vi "InitWaveforms.vi"(6 "First Read":bool, 7 "Samples Per Channel":i32, 8 "error in (no error)":errorcluster, 9 "Sample Rate":dbl, 10 "Units":string[](array[string]), 11 "Channels":string[](array[string])) -> (0 "error out":errorcluster, 3 "wfm array":waveform(sgl)[](array[waveform]))   [LabVIEW 2017, in "cRIOWfmLib.lvlib"]
uses:
  <vilib>/addons/InsightCM/Devices/Shared/Cms/cRIOWfmAcq/cRIOWfmLib.lvlib
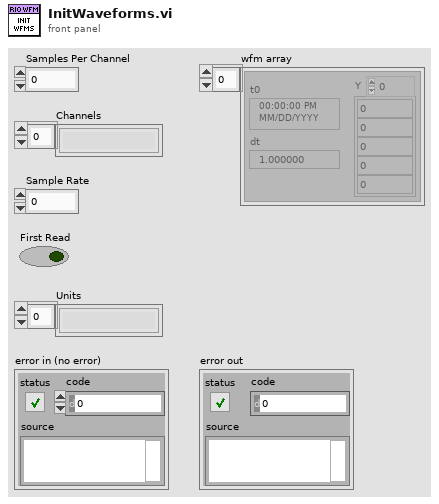
[diagram p1: front panel]
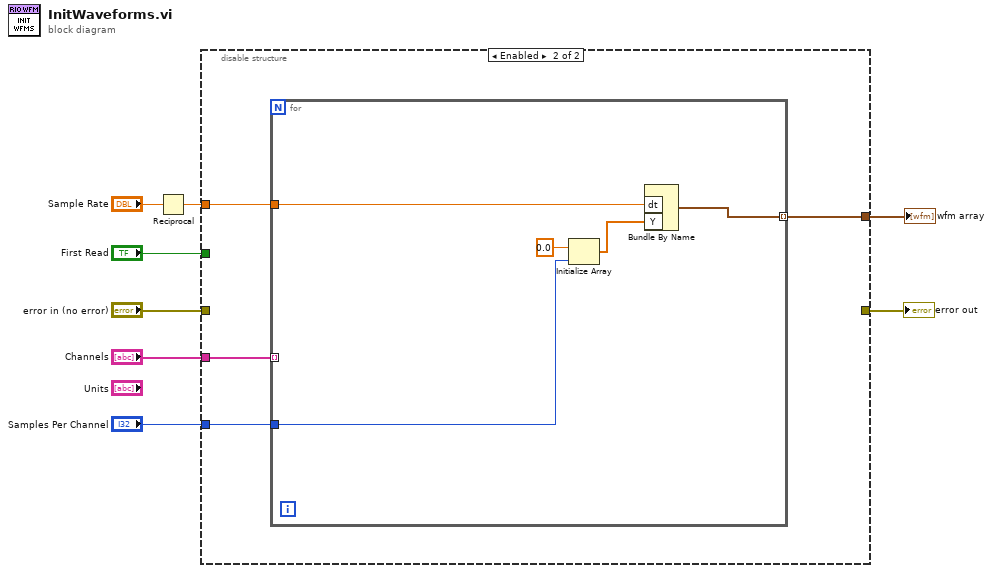
[diagram p0: block diagram]
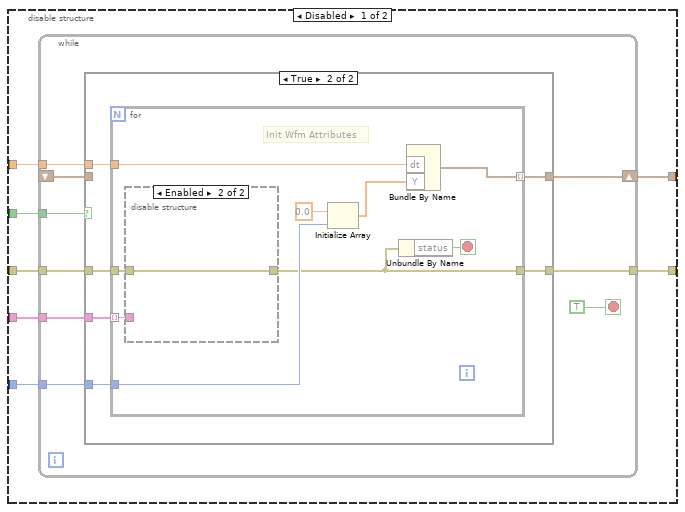
[diagram p2: hidden frame]
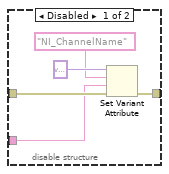
[diagram p4: hidden frame]
diagram:
  n1 = Reciprocal(x="Sample Rate") -> (1/x=w1:dbl)
  n2 = disable-structure shown="Enabled" {
    disable-tunnel: "Samples Per Channel" -> [w15 w49]
    disable-tunnel: "error in (no error)" -> [w14 _]
    disable-tunnel: "First Read" -> [w13 _]
    disable-tunnel: [w12 w48] -> w5
    disable-tunnel: "Channels" -> [w11 w51]
    disable-tunnel: [w10 _] -> w3
    disable-tunnel: w1 -> [w9 w50]
    frame Disabled {
      n3 = while {
        tunnel: w9 -> [w24]
        tunnel: w14 -> [w23]
        tunnel: [w22] -> w10
        tunnel: w11 -> [w21]
        shift-right: [w20] -> w12
        shift-left: _ -> [w18]
        tunnel: w13 -> [w17]
        tunnel: w15 -> [w16]
        stop <- TRUE stop-if-true
        n4 = case shown="True" w17 {
          tunnel: w24 -> [_ w32]
          tunnel: w23 -> [w26 w31]
          tunnel: [w26 w30] -> w22
          tunnel: w21 -> [_ w29]
          tunnel: [w25 w28] -> w20
          tunnel: w18 -> [w25 _]
          tunnel: w16 -> [_ w27]
          frame False {
          }
          frame True {
            n5 = for {
              tunnel: w32 -> [w41]
              tunnel: [w34] -> w28 mode=indexing
              tunnel: w31 -> [w40]
              tunnel: [w33] -> w30
              tunnel: w29 -> [w36] mode=indexing
              tunnel: w27 -> [w37]
              stop <- w39 stop-if-true
              # "Init Wfm Attributes"
              n6 = disable-structure shown="Enabled" {
                disable-tunnel: w40 -> [w46 w47]
                disable-tunnel: w36 -> [w45 _]
                disable-tunnel: [w42 w47] -> w33
                frame Disabled {
                  n7 = Set Variant Attribute(Variant=variant ("variant out"), name="NI_ChannelName", value=w45, error in=w46) -> (error out=w42:errorcluster)  [unwired: 2 out]
                }
                frame Enabled {
                }
              }
              n8 = Initialize Array(sgl 0.0, w37) -> (w35:sgl[])
              n9 = Unbundle By Name(w33) -> ("status"=w39:bool)
              n10 = Bundle By Name("dt"=w41, "Y"=w35) -> (w34:waveform(sgl))  [unwired: 1 out]
            }
          }
        }
      }
    }
    frame Enabled {
      n11 = for {
        tunnel: w51 -> [_] mode=indexing
        tunnel: w50 -> [w56]
        tunnel: w49 -> [w53]
        tunnel: [w52] -> w48 mode=indexing
        n12 = Initialize Array(sgl 0.0, w53) -> (w54:sgl[])
        n13 = Bundle By Name("dt"=w56, "Y"=w54) -> (w52:waveform(sgl))  [unwired: 1 in]
      }
    }
  }
  "wfm array" <- w5
  "error out" <- w3
